vi "Kikusui PLZ-Request.vi"(6 "Response?":bool, 8 "error in":errorcluster, 9 "byte count":u32, 10 "Command":string, 11 "Kikusui PLZ Setting In":T1={"VISA Resource Name"="", "Baud Rate"=19200, "Stop Bits"=20, "Wait For Read(ms)"=0} {"Stop Bits" items=["1.0"=10, "2.0"=20]; "Baud Rate" items=["2400"=2400, "4800"=4800, "9600"=9600, "19200"=19200]}) -> (0 "error out":errorcluster, 2 "Response":string, 3 "Kikusui PLZ Setting Out":T1={"VISA Resource Name"="", "Baud Rate"=19200, "Stop Bits"=20, "Wait For Read(ms)"=0} {"Stop Bits" items=["1.0"=10, "2.0"=20]; "Baud Rate" items=["2400"=2400, "4800"=4800, "9600"=9600, "19200"=19200]})   [LabVIEW 2018]
uses:
  Data Def/Kikusui PLZ-Setting.ctl
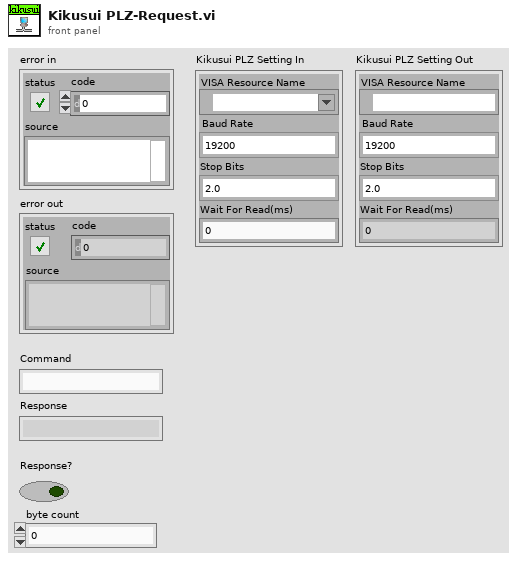
[diagram p1: front panel]
types:
  T1 = typedef "Kikusui PLZ-Setting.ctl" = cluster{"VISA Resource Name":refnum<visa-resource-name>, "Baud Rate":u32, "Stop Bits":u16, "Wait For Read(ms)":u32}
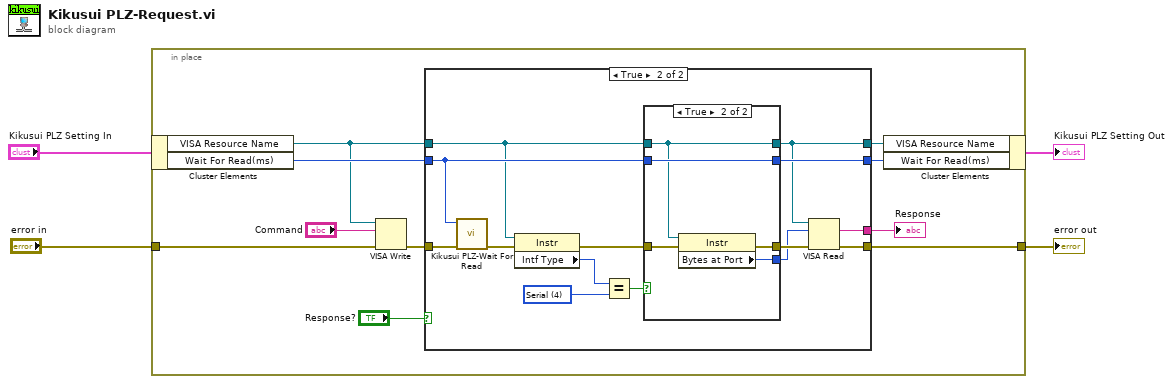
[diagram p0: block diagram]
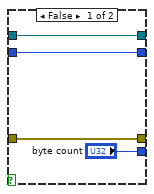
[diagram p3: hidden frame]
diagram:
  n1 = in-place {
    in-place-border: "error in" -> [w13]
    in-place-border: [w10] -> w3
    n2 = in-place-cluster #1("Kikusui PLZ Setting In") -> ("VISA Resource Name"=w8:refnum<visa-resource-name>, "Wait For Read(ms)"=w9:u32)
    n3 = VISA Write(VISA resource name=w8, write buffer="Command", error in (no error)=w13) -> (error out=w12:errorcluster)  [unwired: 2 out]
    n4 = case shown="True" "Response?" {
      tunnel: w12 -> [w17 w31]
      tunnel: [w17 w30] -> w10
      tunnel: w8 -> [w15 w21]
      tunnel: w9 -> [w16 w22]
      tunnel: [w15 w18] -> w7
      tunnel: [w16 w20] -> w6
      tunnel: [_ w19] -> w5
      frame False {
      }
      frame True {
        w28 = u16 4 items=["GPIB"=1, "VXI"=2, "GPIB-VXI"=3, "Serial"=4, "PXI"=5, "TCPIP"=6, "USB"=7] ("Interface Information:Interface Type")
        n5 = call "Kikusui PLZ-Wait For Read.vi"("error in"=w31, "Wait For Read(ms)"=w22) -> ("error out"=w29:errorcluster)  [unwired: 9 in]
        n6 = property class="Instr"(reference=w21, error in=w29) -> (error out=w25:errorcluster, "Intf Type"=w27:u16)  [unwired: 1 out]
        n7 = Equal?(x=w27, y=w28) -> (x = y?=w26:bool)
        n8 = case shown="True" w26 {
          tunnel: w25 -> [w35 w40]
          tunnel: [w35 w39] -> w24
          tunnel: ["byte count" w38] -> w23
          tunnel: w22 -> [w32 w37]
          tunnel: w21 -> [w33 w36]
          tunnel: [w32 w37] -> w20
          tunnel: [w33 w36] -> w18
          frame False {
          }
          frame True {
            n9 = property class="Instr"(reference=w36, error in=w40) -> (error out=w39:errorcluster, "Bytes at Port"=w38:u32)  [unwired: 1 out]
          }
        }
        n10 = VISA Read(VISA resource name=w18, byte count=w23, error in (no error)=w24) -> (read buffer=w19:string, error out=w30:errorcluster)  [unwired: 2 out]
      }
    }
    "Response" <- w5
    n11 = in-place-cluster #1("VISA Resource Name"=w7, "Wait For Read(ms)"=w6) -> (→"Kikusui PLZ Setting Out":T1)
  }
  "error out" <- w3
